vi "SubVI Set Front panel elements.vi"(7 "Enable elements (T)":bool=TRUE, 10 "error in (passthrough)":errorcluster, 11 "Array":refnum<vi>[](array[refnum])) -> (2 "error out":errorcluster)   [LabVIEW 2020, in "QuPMXdriver.lvlib"]
doc: "Set \"Enabled\" or \"Disabled and grayed out\" on elements in reference array."
uses:
  QuPMXdriver.lvlib
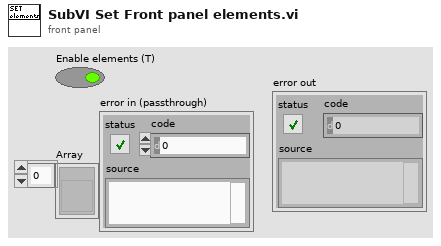
[diagram p1: front panel]
types:
  T1 = enum8{"Enabled", "Disabled", "Disabled and Grayed Out"}
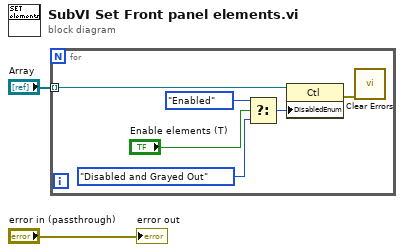
[diagram p0: block diagram]
diagram:
  n1 = for {
    tunnel: "Array" -> [w8] mode=indexing
    n2 = Select(t=T1."Enabled" ("Disabled"), s="Enable elements (T)", f=T1."Disabled and Grayed Out" ("Disabled")) -> (s? t:f=w4:T1)
    n3 = property class="Ctl"(reference=w8, "DisabledEnum"=w4) -> (error out=w3:errorcluster)  [unwired: 1 in, 1 out]
    n4 = call <vilib>:"Clear Errors.vi"("error in (no error)"=w3) -> ()  [unwired: 5 in, 2 out]
  }
  "error out" <- "error in (passthrough)"
